vi "FGV Abort.vi"(8 "error in":errorcluster, 10 "In":bool, 11 "Action":enum16{"Initialize", "Read", "Write"}(ring)) -> (0 "error out":errorcluster, 2 "Out":bool)   [LabVIEW 2019]
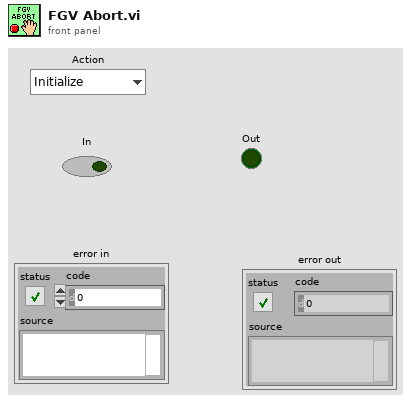
[diagram p1: front panel]
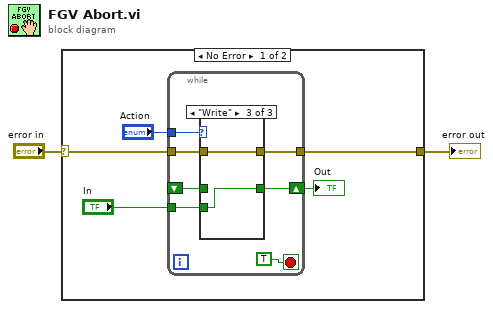
[diagram p0: block diagram]
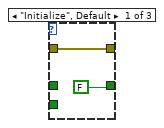
[diagram p2: hidden frame]
diagram:
  n1 = case shown="No Error" "error in" {
    selector: "error in" -> [w6 w21]
    tunnel: [w5 w21] -> w1
    frame No Error {
      n2 = while {
        tunnel: "Action" -> [w14]
        shift-right: [w8] -> w3
        shift-left: _ -> [w12]
        tunnel: "In" -> [w13]
        tunnel: w6 -> [w10]
        tunnel: [w9] -> w5
        stop <- TRUE stop-if-true
        n3 = case shown="\"Write\"" w14 {
          tunnel: w13 -> [_ _ w19]
          tunnel: [FALSE w18 w19] -> w8
          tunnel: w12 -> [_ w18 _]
          tunnel: [w16 w17 w20] -> w9
          tunnel: w10 -> [w16 w17 w20]
          frame "Initialize", Default {
          }
          frame "Read" {
          }
          frame "Write" {
          }
        }
      }
      "Out" <- w3
    }
    frame Error {
    }
  }
  "error out" <- w1
